vi "RSZVB Channel Trace Export Data.vi"(7 "File Name (Trc1.s1p)":string="Trc1.s1p", 8 "error in (no error)":errorcluster {"code" format="%.0x"}, 9 "Channel (Trace) (1)":i32=1, 10 "Select Channel (0: Single)":i32(ring) items=["Single", "All"], 11 "VISA session":refnum<visa-resource-name>) -> (0 "error out":errorcluster {"code" format="%.0x"}, 3 "dup VISA session":refnum<visa-resource-name>)   [LabVIEW 2011]
doc: "This VI stores the trace data of all data traces in the specified channel to a trace file.\n\nNote(s):\n\nTraces are created using the CALCulte<Ch>:PARameter:SDEFine... command.\n\n*.s<n>p Touchstone files (<n> = 1, 2, 3, ...) are intended for a complete set of <n>-port S-parameters. Data export fails if the active channel does not contain the full set of <n>^2 traces. \n\n\nRemote-control command(s):\nMMEMory:STORe:TRACe:CHANnel <ch_number> | ALL,'<file_name>'"
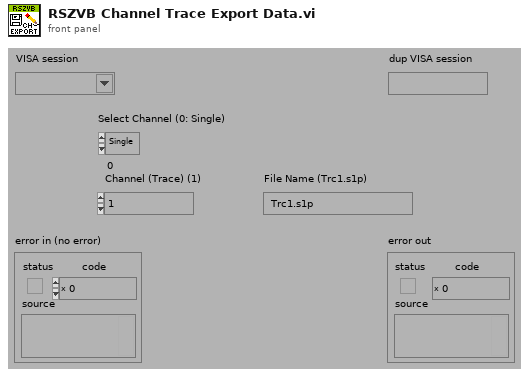
[diagram p1: front panel]
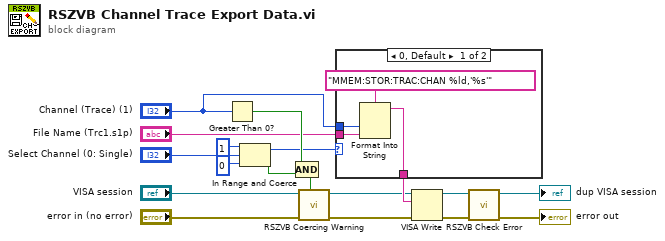
[diagram p0: block diagram]
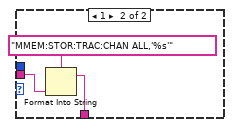
[diagram p2: hidden frame]
diagram:
  n1 = Greater Than 0?(x="Channel (Trace) (1)") -> (x > 0?=w10:bool)
  n2 = In Range and Coerce(upper limit=1, x="Select Channel (0: Single)", lower limit=0) -> (coerced(x)=w3:i32, In Range?=w12:bool)
  n3 = Compound Arithmetic op=AND(w10, w12) -> (w15:bool)
  n4 = call "RSZVB Coercing Warning.vi"("In Range?"=w15, "error in (no error)"="error in (no error)", "VISA session"="VISA session") -> ("error out"=w7:errorcluster, "dup VISA session"=w6:refnum<visa-resource-name>)  [unwired: 7 in]
  n5 = case shown="0, Default" w3 {
    tunnel: [w22 w24] -> w16
    tunnel: "Channel (Trace) (1)" -> [w20 _]
    tunnel: "File Name (Trc1.s1p)" -> [w19 w23]
    frame 0, Default {
      n6 = Format Into String(format string="MMEM:STOR:TRAC:CHAN %ld,'%s'", w20, w19) -> (resulting string=w22:string)  [unwired: 2 in, 1 out]
    }
    frame 1 {
      n7 = Format Into String(format string="MMEM:STOR:TRAC:CHAN ALL,'%s'", w23) -> (resulting string=w24:string)  [unwired: 2 in, 1 out]
    }
  }
  n8 = VISA Write(VISA resource name=w6, write buffer=w16, error in (no error)=w7) -> (VISA resource name out=w17:refnum<visa-resource-name>, error out=w18:errorcluster)  [unwired: 1 out]
  n9 = call "RSZVB Check Error.vi"("error in (no error)"=w18, "VISA session"=w17) -> ("error out"=→"error out":errorcluster, "dup VISA session"=→"dup VISA session":refnum<visa-resource-name>)  [unwired: 8 in]
